vi "PE7260_readout.vi"(2 "mode":dbl, 3 "delay time":dbl, 4 "address":string) -> (0 "7265 Y":dbl format="%#_14g", 1 "7265 X":dbl format="%#_14g")   [LabVIEW 2018]
uses:
  Instrument_Setup.vi
panel:
  out "7265 Y (V)":string="1.298E-05\r\n"
  out "7265 X (V)":string="1.298E-05\r\n"
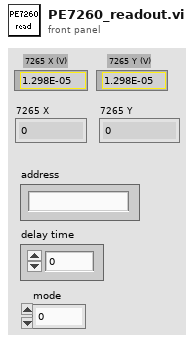
[diagram p1: front panel]
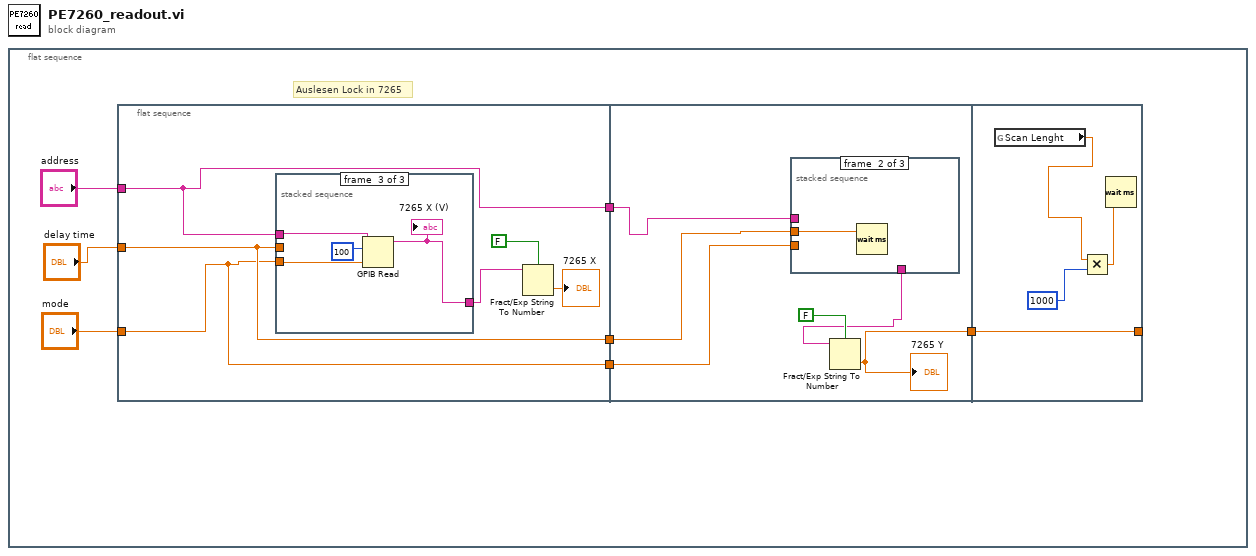
[diagram p0: block diagram]
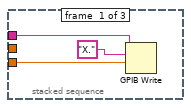
[diagram p2: hidden frame]
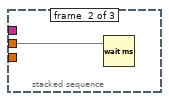
[diagram p3: hidden frame]
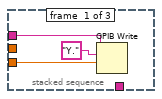
[diagram p4: hidden frame]
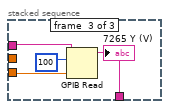
[diagram p5: hidden frame]
diagram:
  n1 = flat-sequence {
    frame #0 {
      # "Auslesen Lock in 7265"
      n2 = flat-sequence {
        tunnel: [w10] -> w7
        tunnel: "address" -> [w10]
        tunnel: "delay time" -> [w9]
        tunnel: "mode" -> [w8]
        tunnel: [w9] -> w2
        tunnel: [w8] -> w1
        tunnel: w7 -> [w24]
        tunnel: [w25] -> w6
        tunnel: w2 -> [w23]
        tunnel: w1 -> [w22]
        tunnel: [w39] -> _
        tunnel: w6 -> [w39]
        frame #0 {
          n3 = stacked-sequence {
            tunnel: w10 -> [w16 _ w20]
            tunnel: w8 -> [w15 _ w21]
            tunnel: w9 -> [_ w17 _]
            tunnel: [_ _ w19] -> w12
            frame #0 {
              n4 = GPIB Write(0:w16, 1:"X.", 2:w15) -> ()  [unwired: 2 in, 2 out]
            }
            frame #1 {
              n5 = Wait (ms)(milliseconds to wait=w17) -> ()  [unwired: 1 out]
            }
            frame #2 {
              n6 = GPIB Read(0:w20, 1:100, 2:w21) -> (5:w19:string)  [unwired: 2 in, 2 out]
              "7265 X (V)" <- w19
            }
          }
          n7 = Fract/Exp String To Number(use system decimal point (T)=FALSE, string=w12) -> (number=→"7265 X":dbl)  [unwired: 2 in, 1 out]
        }
        frame #1 {
          n8 = stacked-sequence {
            tunnel: w24 -> [w30 _ w34]
            tunnel: w22 -> [w29 _ w35]
            tunnel: w23 -> [_ w31 _]
            tunnel: [_ _ w33] -> w26
            frame #0 {
              n9 = GPIB Write(0:w30, 1:"Y.", 2:w29) -> ()  [unwired: 2 in, 2 out]
            }
            frame #1 {
              n10 = Wait (ms)(milliseconds to wait=w31) -> ()  [unwired: 1 out]
            }
            frame #2 {
              n11 = GPIB Read(0:w34, 1:100, 2:w35) -> (5:w33:string)  [unwired: 2 in, 2 out]
              "7265 Y (V)" <- w33
            }
          }
          n12 = Fract/Exp String To Number(use system decimal point (T)=FALSE, string=w26) -> (number=w25:dbl)  [unwired: 2 in, 1 out]
          "7265 Y" <- w25
        }
        frame #2 {
          n13 = global read "Instrument_Setup.vi" "Scan Lenght"() -> (w36:dbl)
          n14 = Multiply(x=w36, y=1000) -> (x*y=w37:dbl)
          n15 = Wait (ms)(milliseconds to wait=w37) -> ()  [unwired: 1 out]
        }
      }
    }
  }
